vi "DAC Init Results.vi"(8 "error in":errorcluster, 9 "Log Details?":bool, 10 "tdms file":refnum<k34>, 11 "DAC Pump Inv in":refnum<class "DAC Pump Inv.lvclass">) -> (0 "error out":errorcluster, 2 "tdms file out":refnum<k34>)   [LabVIEW 2019, in "DAC.lvlib" / "DAC Pump Inv.lvclass"]
uses:
  DAC Pump Inv.lvclass
  C:/Users/wg/Documents/LV_Projects/test-stand/App/DAC/DAC.lvclass
  DAC.lvclass/DAC.ctl
  DAC Pump Inv.lvclass/DAC Pump Inv.ctl
  DAC.lvclass
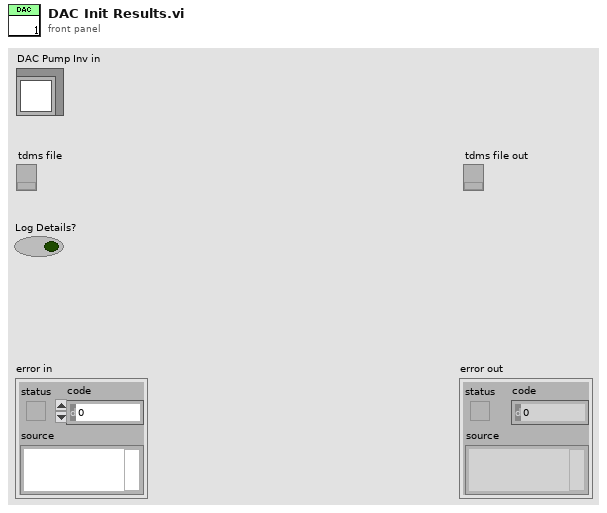
[diagram p1: front panel]
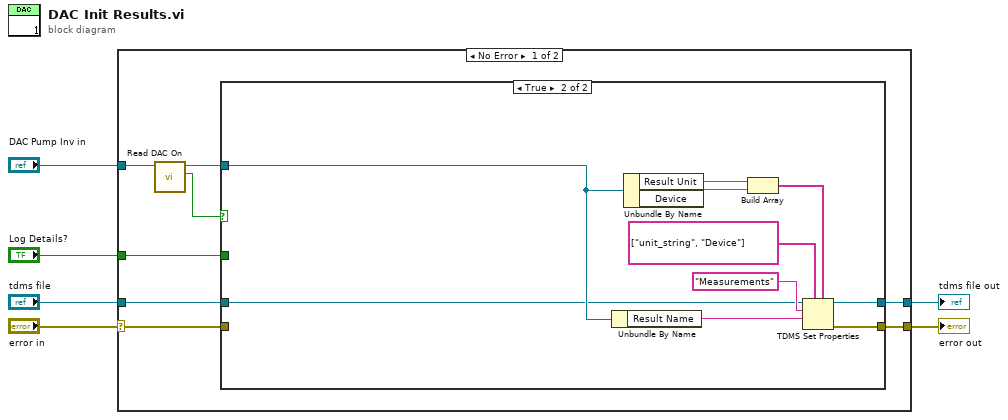
[diagram p0: block diagram]
diagram:
  n1 = case shown="No Error" "error in" {
    selector: "error in" -> [w10 w28]
    tunnel: [w7 w28] -> w6
    tunnel: "DAC Pump Inv in" -> [w14 _]
    tunnel: "tdms file" -> [w11 w27]
    tunnel: [w8 w27] -> w5
    tunnel: "Log Details?" -> [w9 _]
    frame No Error {
      n2 = call "Read DAC On.vi"("DAC in"=w14) -> ("DAC On"=w12:bool, "DAC out"=w13:refnum<class "DAC Pump Inv.lvclass">)  [unwired: 8 in, 1 out]
      n3 = case shown="True" w12 {
        tunnel: w11 -> [w15 w17]
        tunnel: [w15 w19] -> w8
        tunnel: [w16 w20] -> w7
        tunnel: w13 -> [_ w18]
        tunnel: w10 -> [w16 _]
        tunnel: w9 -> [_ _]
        frame False {
        }
        frame True {
          n4 = Unbundle By Name(w18) -> ("Result Name"=w22:string)
          n5 = Unbundle By Name(w18) -> ("Result Unit"=w24:string, "Device"=w21:string)
          n6 = Build Array(w24, w21) -> (w23:string[])
          n7 = TDMS Set Properties(5:w23, 7:string[] ["unit_string", "Device"] ("property names"), 9:w22, 10:"Measurements" ("group name in (Untitled)"), 11:w17) -> (0:w20:errorcluster, 3:w19:refnum<k34>)  [unwired: 1 in, 2 out]
        }
      }
    }
    frame Error {
    }
  }
  "error out" <- w6
  "tdms file out" <- w5
